vi "Value.vi"(8 "Error In":errorcluster, 11 "Number Widget In":refnum<class "6. Number Widget.lvclass">) -> (0 "Error Out":errorcluster, 2 "Value":dbl, 3 "Number Widget Out":refnum<class "6. Number Widget.lvclass">)   [LabVIEW 2013, in "6. Number Widget.lvclass"]
uses:
  6. Number Widget.lvclass
  6. Number Widget.lvclass/6. Number Widget.ctl
  src/LabVIEW/Qwt/QwtAbstractSlider/QwtAbstractSlider.lvclass
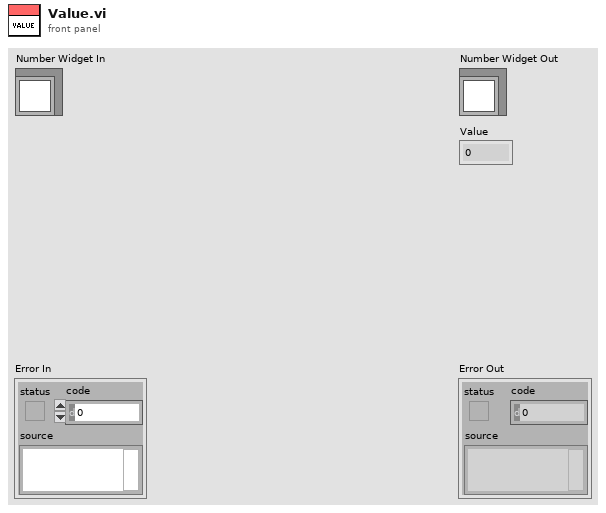
[diagram p1: front panel]
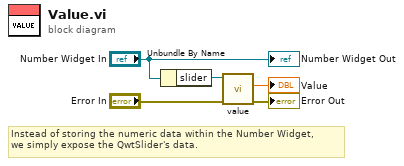
[diagram p0: block diagram]
diagram:
  # "Instead of storing the numeric data within the Number Widget,\nwe simply expose the QwtSlider's data."
  n1 = Unbundle By Name("Number Widget In") -> ("slider"=w4:refnum<class "QwtSlider.lvclass">)
  n2 = call "value.vi"("Error In"="Error In", "QwtAbstractSlider In"=w4) -> ("Error Out"=→"Error Out":errorcluster, "Value"=→"Value":dbl)  [unwired: 7 in, 1 out]
  "Number Widget Out" <- "Number Widget In"
